vi "PH_Synchrolock_Watch.set modified data.vi"(0 "i ref in":refnum<vi>, 2 "i attribute":T1={"GUI Refs"={"Mean Phase Graph"=refnum, "RF Amplitude Graph"=refnum, "Mira Amplitude Graph"=refnum, "MIRA State"=refnum, "Mean Phase"=refnum, "RF Amplitude"=refnum, "Mira Amplitude"=refnum, "Mean Phase in range?"=refnum, "RF Amplitude above limit?"=refnum, "Mira Amplitude in range?"=refnum, "Mean phase upper limit"=refnum, "Mean phase lower limit"=refnum, "RF Amplitude lower limit"=refnum, "Mira Amplitude lower limit"=refnum, "Mira Amplitude upper limit"=refnum, "Waveform End"=refnum, "Mira scope"=refnum, "Reset Mira warning"=refnum}, "Status"={"Reset Warning"=FALSE}, "Mean Phase"={"Current Value"=0.0, "Upper Limit"=0.0, "Lower Limit"=0.0, "Data"={[], []}}, "RF"={"Current Value"=0.0, "Lower Limit"=0.0, "Data"={[], []}}, "MIRA"={"Current Value"=0.0, "Upper Limit"=0.0, "Lower Limit"=0.0, "Data"={[], []}}, "Waveform End"=10000}, 5 "error in (no error)":errorcluster) -> (14 "i ref out":refnum<vi>, 19 "error out":errorcluster)   [LabVIEW 2014, in "PH_Synchrolock_Watch.lvlib"]
doc: "Writes the data into the attribute of an object. Then, the attribute dara are unlocked using the \"release\" method. Prior to calling THIS method, the attribute data must have been locked using the methods \"lock\" or \"get data to modify\".\n\n\nLicense Agreement for this software:\n\nCopyright (C)\nGesellschaft für Schwerionenforschung, GSI\nPlanckstr. 1\n64291 Darmstadt\nGermany\n\nContact: D.Beck@gsi.de \n\nThis program is free software; you can redistribute it and/or modify it under the terms of the GNU General Public License as published by the Free Software Foundation; either version 2 of the license, or (at your option) any later version.\n\nThis program is distributed in the hope that it will be useful, but WITHOUT ANY WARRANTY; without even the implied warranty of MERCHANTABILITY or FITNESS FOR A PARTICULAR PURPOSE. See the GNU General License for more details (http://www.gnu.org).\n\nGesellschaft für Schwerionenforschung, GSI\nPlanckstr. 1, 64291 Darmstadt, Germany\nFor all questions and ideas contact: M.Richter@gsi.de, H.Brand@gsi.de or D.Beck@gsi.de.\nLast update: 17-JUN-2004"
uses:
  PH_Synchrolock_Watch.lvlib
  PH_Synchrolock_Watch.i attribute.ctl
  CS_Core/CSObj/CSObj.lvlib
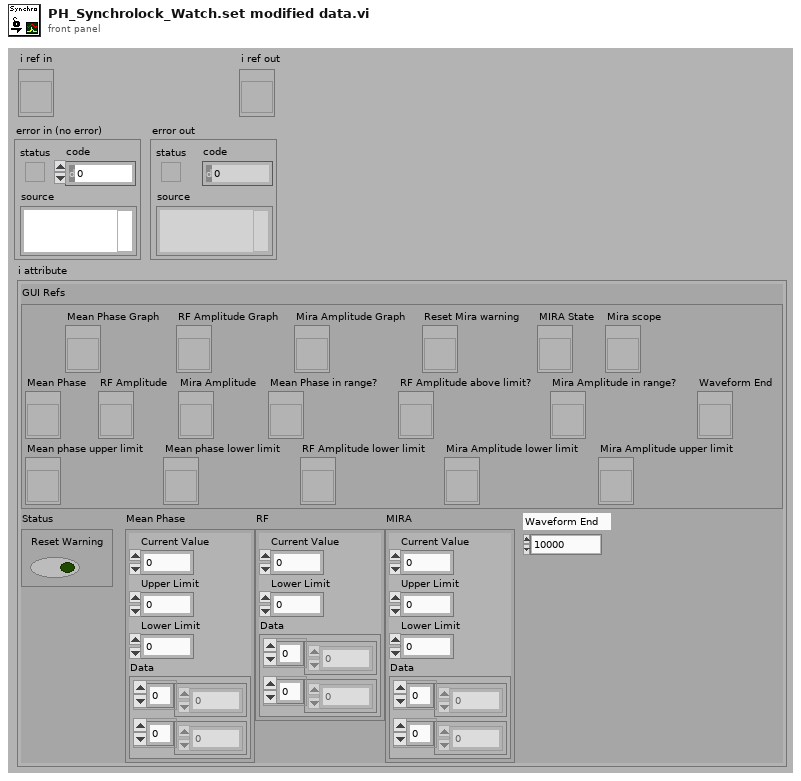
[diagram p1: front panel]
types:
  T1 = typedef "PH_Synchrolock_Watch.lvlib/PH_Synchrolock_Watch.i attribute.ctl" = cluster{"GUI Refs":cluster{"Mean Phase Graph":refnum<vi>, "RF Amplitude Graph":refnum<vi>, "Mira Amplitude Graph":refnum<vi>, "MIRA State":refnum<vi>, "Mean Phase":refnum<vi>, "RF Amplitude":refnum<vi>, "Mira Amplitude":refnum<vi>, "Mean Phase in range?":refnum<vi>, "RF Amplitude above limit?":refnum<vi>, "Mira Amplitude in range?":refnum<vi>, "Mean phase upper limit":refnum<vi>, "Mean phase lower limit":refnum<vi>, "RF Amplitude lower limit":refnum<vi>, "Mira Amplitude lower limit":refnum<vi>, "Mira Amplitude upper limit":refnum<vi>, "Waveform End":refnum<vi>, "Mira scope":refnum<vi>, "Reset Mira warning":refnum<vi>}, "Status":cluster{"Reset Warning":bool}, "Mean Phase":cluster{"Current Value":dbl, "Upper Limit":dbl, "Lower Limit":dbl, "Data":cluster{dbl[], dbl[]}}, "RF":cluster{"Current Value":dbl, "Lower Limit":dbl, "Data":cluster{dbl[], dbl[]}}, "MIRA":cluster{"Current Value":dbl, "Upper Limit":dbl, "Lower Limit":dbl, "Data":cluster{dbl[], dbl[]}}, "Waveform End":i32}
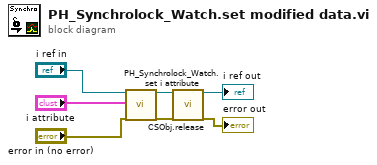
[diagram p0: block diagram]
diagram:
  n1 = call "PH_Synchrolock_Watch.set i attribute.vi"("i ref in"="i ref in", "i attribute"="i attribute", "error in (no error)"="error in (no error)") -> ("i ref out"=w4:refnum<vi>, "error out"=w3:errorcluster)  [unwired: 15 in]
  n2 = call "CSObj.release.vi"("i ref in"=w4, "error in (no error)"=w3) -> ("i ref out"=→"i ref out":refnum<vi>, "error out"=→"error out":errorcluster)  [unwired: 16 in]
